vi "Global.vi"() -> ()   [LabVIEW 2017, in "Ballard Arinc-429 Shared.lvlib"]
uses:
  Ballard Arinc-429 Shared.lvlib
panel:
  in  "Tx Config":string="Tx Config"
  in  "Rx Config":string="Rx Config"
  in  "WordInitialRawValue":string="WordInitialRawValue"
  in  "Load Database - Message1":string="Warning. At least another Custom Device instance is configured with same Hardware Configuration File. It is a supported use-case and more for user's attention."
  in  "On Save Action VI - Message1":string="Error. Several Arinc-429 Ballard Custom Device instances have same combination of Card and Core Number. Deployment won't complete successfully."
  in  "Encoding Type":string="Encoding Type"
  in  "Unit":string="Unit"
  in  "Load Parameters File Action VI - Message2":string="There is already a Parameters File loaded. Click OK to continue and all existing System Mappings (connecting Parameters Channels) will be lost. Click Cancel to stop load operation."
  in  "ParametersFileHash":string="ParametersFileHash"
  in  "Load Parameters File Action VI - Message1":string="There is no Hardware Configuration loaded. You cannot load a Parameters File."
  in  "Win Parameters File Path":string="Win Parameters File Path"
  in  "RawData Bits":string="RawData Bits"
  in  "card number":string="card number"
  in  "core number":string="core number"
  in  "Timestamp Channel GUID (default)":string="03D3BB99-1485-13A6-561D1F898F032919"
  in  "bufferSize":string="bufferSize"
  in  "TransferType":string="TransferType"
  in  "Word Section Page GUID":string="f8b859b6-d72b-4d9b-b1ec-c93bcf5b4a07"
  in  "ScheduledSDI":string="ScheduledSDI"
  in  "xmlName":string="xmlName"
  in  "SDIValue":string="SDIValue"
  in  "SDI_Enabled":string="SDI_Enabled"
  in  "ScaleOffset":string="ScaleOffset"
  in  "ScaleFac":string="ScaleFac"
  in  "Signed?":string="Signed?"
  in  "txRate":string="txRate"
  in  "DBHash":string="DBHash"
  in  "WinBinCache":string="Temp429BinFiles"
  in  "MainDisabled":string="7a14808d-e851-4795-811f-53a08b4e5e78"
  in  "MainEnabled":string="dcf168dc-a9fa-4dd1-862e-68da37a31a51"
  in  "InputsReadRate":string="InputsReadRate"
  in  "LoopTime":string="Loop Time"
  in  "OutLoopTime":string="Outputs Loop Duration"
  in  "Status Section":string="Status"
  in  "Error Code":string="Error Code"
  in  "HWIn Late Count":string="Inputs Late Count"
  in  "HWOut Late Count":string="Outputs Late Count"
  in  "Static Chan GUID":string="2c3aa894-526f-4c66-b57e-ee49cdf07fbc"
  in  "Default word":string="Default word"
  in  "Status Section GUID":string="3ca1cf51-256d-4b71-b262-84a241d665fd"
  in  "Num Bits":string="Num Bits"
  in  "Channel Page GUID":string="308ffbea-fdbc-4ce1-9e62-f3cbc8f02371"
  in  "Channel #":string="Channel #"
  in  "HWOutputs GUID":string="ff22a48e-3d72-4582-973e-954b49f921ff"
  in  "HWInputs GUID":string="7d9e3a61-fe41-466b-9522-b9b7b1585e41"
  in  "Win File Path":string="Win File Path"
  in  "Start Bit":string="Start Bit"
  in  "RT File Path":string="RT File Path"
  in  "Type":string="Type"
  in  "Outputs":string="Outputs - Tx"
  in  "Inputs":string="Inputs - Rx"
  in  "transferPeriod":string="transferPeriod"
  in  "Label Section Page GUID":string="65bb7e5d-e74d-4d35-8b5b-b366e9e62c9b"
  in  "Label Data Page GUID":string="fc1a8733-ba52-4655-a0d0-1a549ed3f86b"
  in  "Label":string="Label"
  # "6de686c8-271d-4eac-aefc-5952b5c6028a"
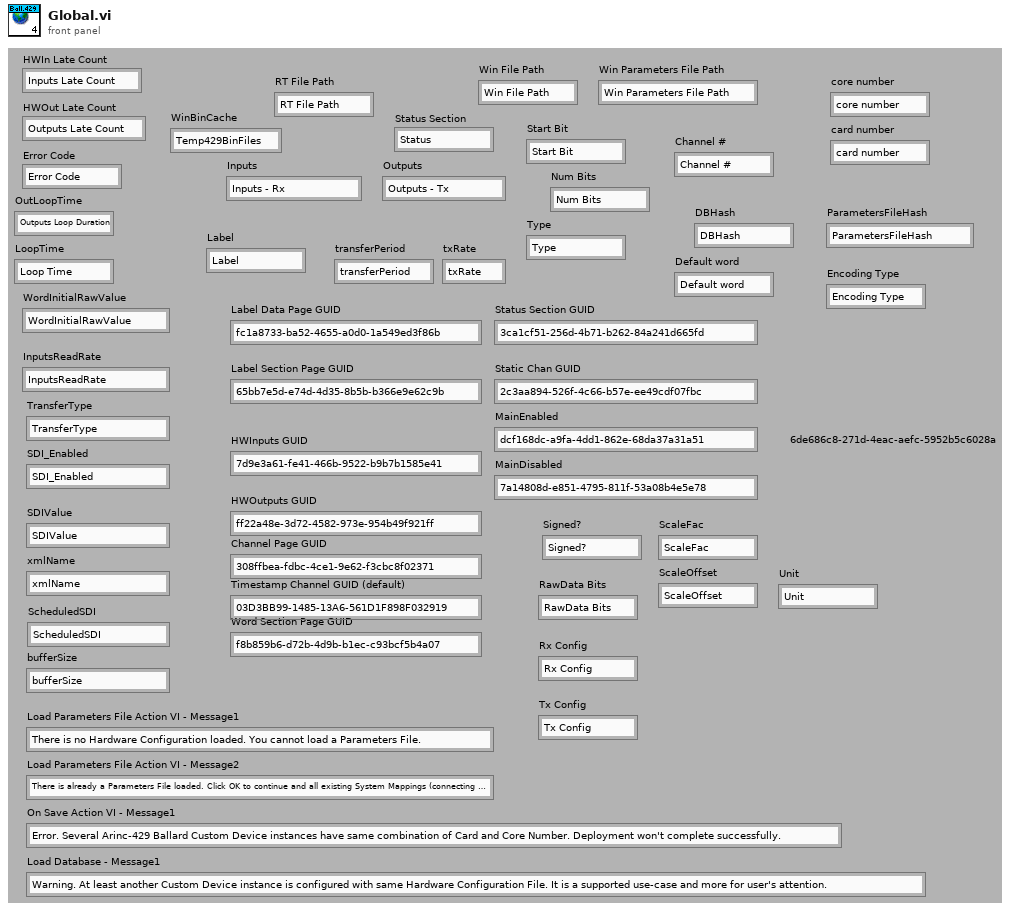
[diagram p1: front panel]
diagram:
